vi "IMAQ Enumerate Cameras.vi"(8 "error in":errorcluster) -> (0 "error out":errorcluster, 3 "IMAQ Interfaces":string[](array[string]))   [LabVIEW 2011]
doc: "This VI allows you to enumerate any IMAQ interfaces (cameras) that are pre-configured in Measurement & Automation Explorer (MAX). If the correct camera or settings are not configured correctly in MAX they will need to be configured correctlythere before this VI will be useful."
panel:
  out "error out 2":errorcluster
  out "Array":string[](array[string])
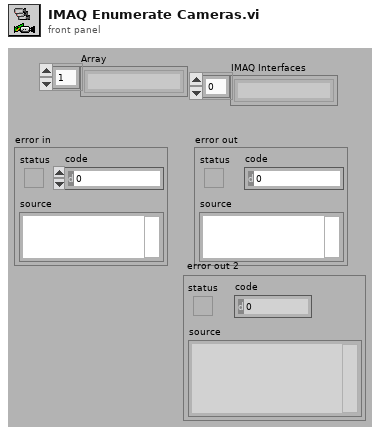
[diagram p1: front panel]
types:
  T1 = typedef "IMAQ Image.ctl" = refnum<image>
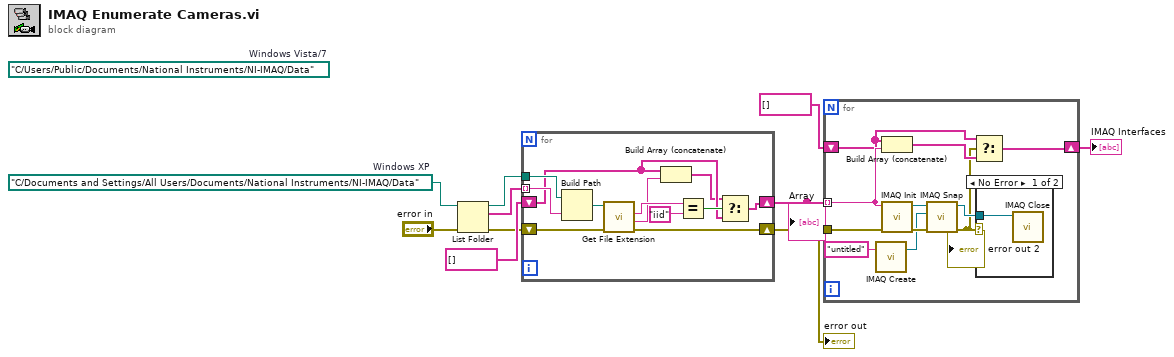
[diagram p0: block diagram]
diagram:
  (unwired) path "C:/Users/Public/Documents/National Instruments/NI-IMAQ/Data"  # Windows Vista/7
  w1 = path "C:/Documents and Settings/All Users/Documents/National Instruments/NI-IMAQ/Data"  # Windows XP
  n1 = List Folder(path=w1, error in="error in") -> (path out=w10:path, filenames=w9:string[], error out=w6:errorcluster)  [unwired: 2 in, 1 out]
  n2 = for {
    tunnel: w9 -> [w21] mode=indexing
    tunnel: w10 -> [w22]
    shift-right: [w16] -> w7
    shift-left: string[] [] -> [w15]
    shift-right: [w11] -> w2
    shift-left: w6 -> [w12]
    n3 = Build Path(base path=w22, name or relative path=w21) -> (appended path=w20:path)
    n4 = call <vilib>:"Get File Extension.vi"("error in (no error)"=w12, "file"=w20) -> ("error out"=w11:errorcluster, "filename without extension"=w14:string, "lowercase file extension"=w19:string)  [unwired: 6 in, 1 out]
    n5 = Build Array (concatenate)(w15, w14) -> (w13:string[])
    n6 = Equal?(x=w19, y="iid") -> (x = y?=w17:bool)
    n7 = Select(t=w13, s=w17, f=w15) -> (s? t:f=w16:string[])
  }
  "error out" <- w2
  "Array" <- w7
  n8 = for {
    tunnel: w7 -> [w32] mode=indexing
    tunnel: w2 -> [w33]
    shift-right: [w29] -> w3
    shift-left: string[] [] -> [w30]
    n9 = call "IMAQ Create"("Image Name"="untitled") -> ("New Image"=w25:T1)  [unwired: 3 in, 2 out]
    n10 = Build Array (concatenate)(w30, w32) -> (w31:string[])
    n11 = call <vilib>:"IMAQ Init.vi"("error in (no error)"=w33, "Interface Name"=w32) -> ("error out"=w26:errorcluster, "IMAQ Session Out"=w28:refnum<k11>)  [unwired: 8 in]
    n12 = call <vilib>:"IMAQ Snap.vi"("error in (no error)"=w26, "Image In"=w25, "IMAQ Session In"=w28) -> ("error out"=w23:errorcluster, "IMAQ Session Out"=w27:refnum<k11>)  [unwired: 6 in, 1 out]
    "error out 2" <- w23
    n13 = Select(t=w30, s=w23, f=w31) -> (s? t:f=w29:string[])
    n14 = case shown="No Error" w23 {
      tunnel: w27 -> [w34 _]
      frame No Error {
        n15 = call <vilib>:"IMAQ Close.vi"("IMAQ Session In"=w34) -> ()  [unwired: 10 in, 1 out]
      }
      frame Error {
      }
    }
  }
  "IMAQ Interfaces" <- w3
